vi "Open List To Inconsistent List.vi"(11 "AD* in":refnum<class "NI_Robotics_AnytimeDStar.lvclass">) -> (3 "AD* out":refnum<class "NI_Robotics_AnytimeDStar.lvclass">)   [LabVIEW 2017, in "NI_Robotics_AnytimeDStar.lvclass"]
uses:
  <vilib>/robotics/Navigation/Anytime D Star/NI_Robotics_AnytimeDStar.lvclass
  <vilib>/robotics/Navigation/Anytime D Star/NI_Robotics_AnytimeDStar.lvclass/NI_Robotics_AnytimeDStar.ctl
  <vilib>/robotics/Navigation/shared/MapNode/AbstractDstarNode/NI_Robotics_AbstractDstarNode.lvclass
  <vilib>/robotics/Navigation/shared/Priority Queue/NI_Robotics_Priority Queue.lvclass
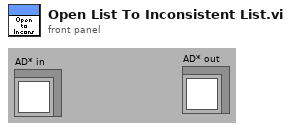
[diagram p1: front panel]
types:
  T1 = typedef "NI_Robotics_Priority Queue.lvclass/Open List Element.ctl" = cluster{"f":dbl, "g":dbl, "node Ref":refnum<data-value>}
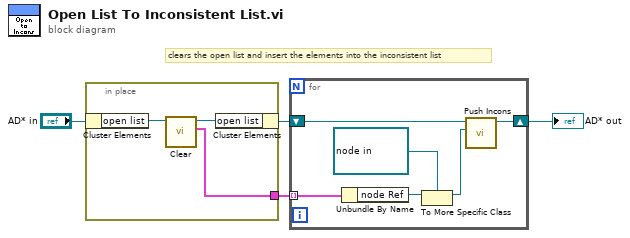
[diagram p0: block diagram]
diagram:
  # "clears the open list and insert the elements into the inconsistent list"
  n1 = in-place {
    in-place-border: [w5] -> w2
    n2 = in-place-cluster #1("AD* in") -> ("open list"=w7:refnum<class "NI_Robotics_Priority Queue.lvclass">)
    n3 = call <vilib>:"Clear.vi"("Priority Queue in"=w7) -> ("Open List"=w5:T1[], "Priority Queue out"=w6:refnum<class "NI_Robotics_Priority Queue.lvclass">)  [unwired: 8 in, 1 out]
    n4 = in-place-cluster #1("open list"=w6) -> (w3:refnum<class "NI_Robotics_AnytimeDStar.lvclass">)
  }
  n5 = for {
    tunnel: w2 -> [w12] mode=indexing
    shift-right: [w13] -> w1
    shift-left: w3 -> [w8]
    n6 = Unbundle By Name(w12) -> ("node Ref"=w10:refnum<data-value>)
    n7 = To More Specific Class(target class=refnum<data-value> refnum ("node ref in"), reference=w10) -> (specific class reference=w9:refnum<data-value>)  [unwired: 1 in, 1 out]
    n8 = call <vilib>:"Push Incons.vi"("node ref in"=w9, "adstar in"=w8) -> ("adstar out"=w13:refnum<class "NI_Robotics_AnytimeDStar.lvclass">)  [unwired: 8 in, 1 out]
  }
  "AD* out" <- w1
